vi "SeCrTs-Drive_Read_L.vi"(8 "error in":errorcluster, 9 "Message Queue":refnum<queue>, 11 "Data FIFO Ref":T1) -> (0 "error out":errorcluster)   [LabVIEW 2022 SP3]
uses:
  RT Controls/SeCrTs-Data FIFO.ctl
  RT Support/SeCrTs-RT_Global_R.vi
panel:
  in  "TCP_Port_Bottom":u16=3000
  in  "TCP_Port_Top":u16=2000
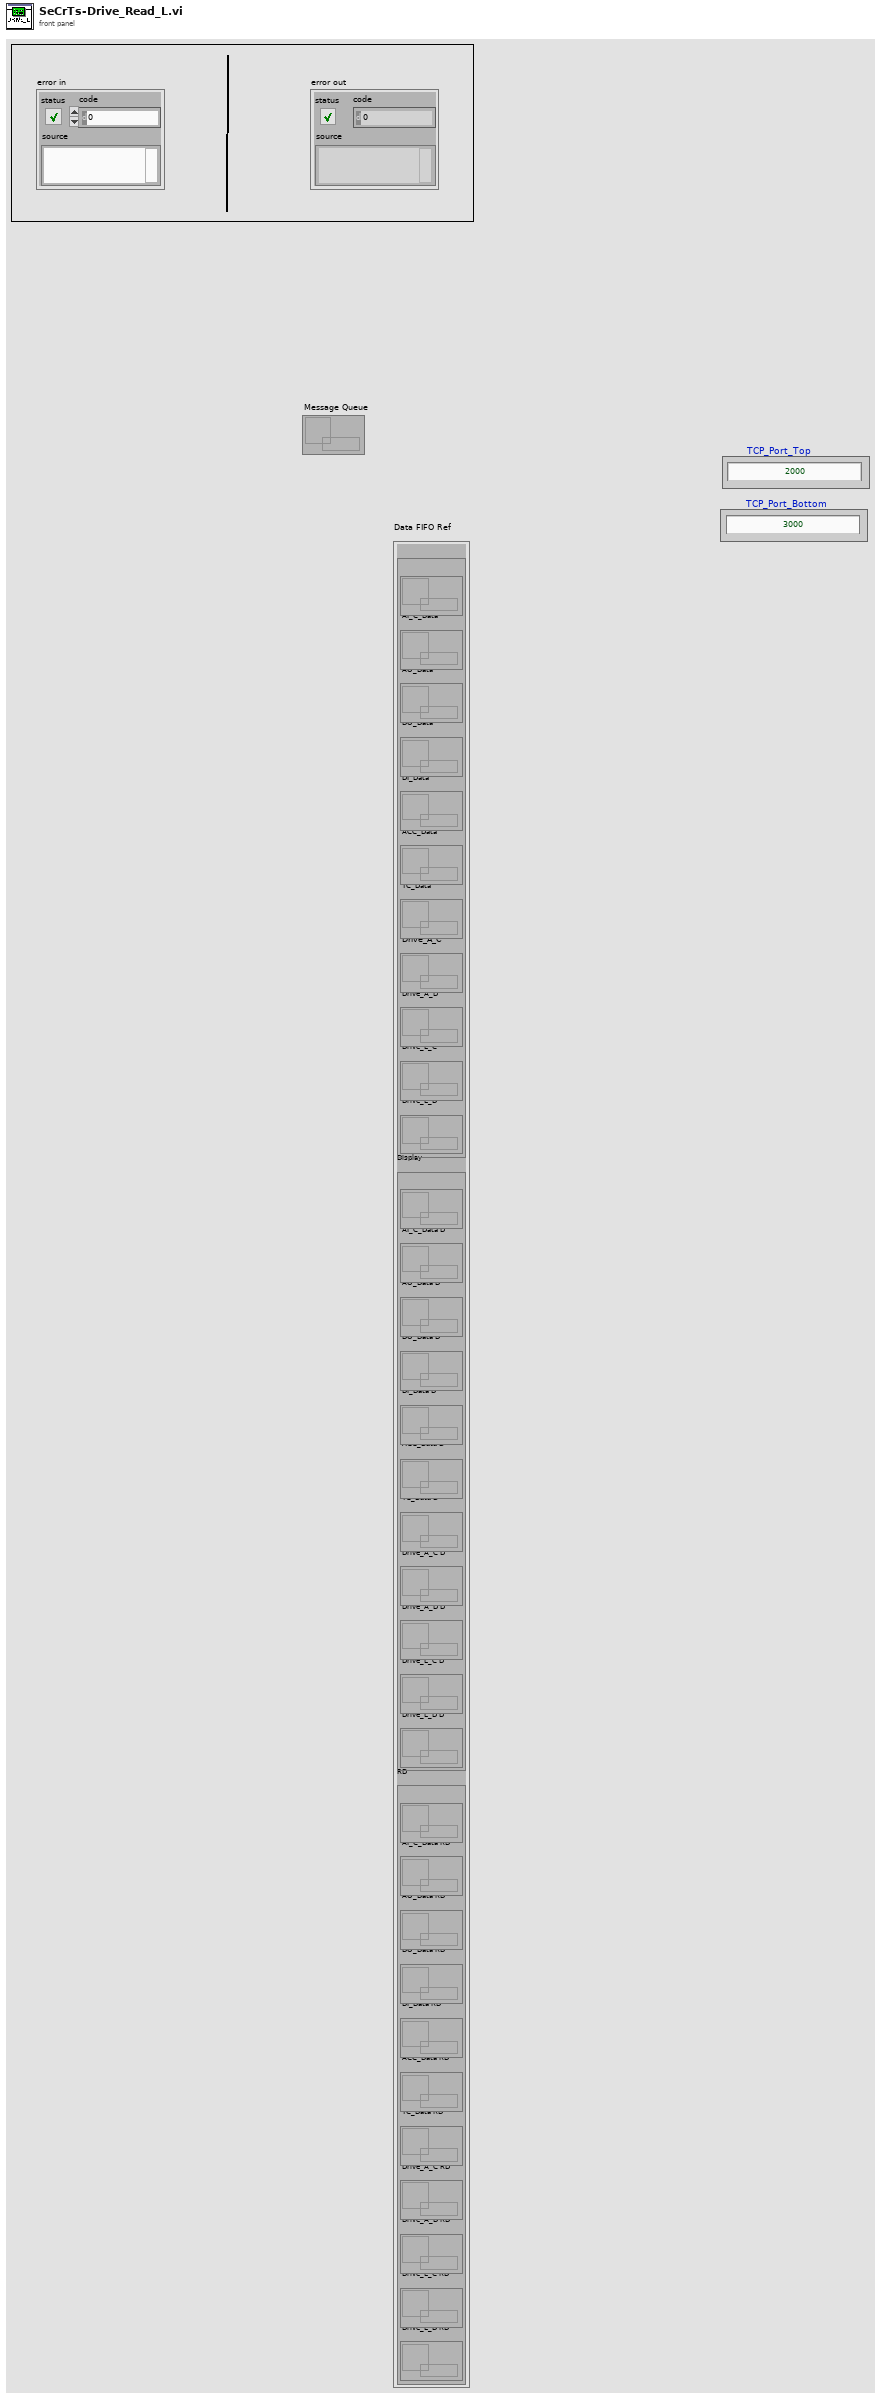
[diagram p1: front panel]
types:
  T1 = typedef "SeCrTs-Data FIFO.ctl" = cluster{"Control":cluster{"AI_V_Data":refnum<queue>, "AI_C_Data":refnum<queue>, "AO_Data":refnum<queue>, "DO_Data":refnum<queue>, "DI_Data":refnum<queue>, "ACC_Data":refnum<queue>, "TC_Data":refnum<queue>, "Drive_A_C":refnum<queue>, "Drive_A_D":refnum<queue>, "Drive_L_C":refnum<queue>, "Drive_L_D":refnum<queue>}, "Display":cluster{"AI_V_Data D":refnum<queue>, "AI_C_Data D":refnum<queue>, "AO_Data D":refnum<queue>, "DO_Data D":refnum<queue>, "DI_Data D":refnum<queue>, "ACC_Data D":refnum<queue>, "TC_Data D":refnum<queue>, "Drive_A_C D":refnum<queue>, "Drive_A_D D":refnum<queue>, "Drive_L_C D":refnum<queue>, "Drive_L_D D":refnum<queue>}, "RD":cluster{"AI_V_Data RD":refnum<queue>, "AI_C_Data RD":refnum<queue>, "AO_Data RD":refnum<queue>, "DO_Data RD":refnum<queue>, "DI_Data RD":refnum<queue>, "ACC_Data RD":refnum<queue>, "TC_Data RD":refnum<queue>, "Drive_A_C RD":refnum<queue>, "Drive_A_D RD":refnum<queue>, "Drive_L_C RD":refnum<queue>, "Drive_L_D RD":refnum<queue>}}
  T2 = enum16{"AI C", "AI V", "AO", "DI", "DO", "TC", "ACC", "DR L", "DR A"}
  T3 = enum16{"Init", "Read 'All'", "Read 'n'", "Read '1'", "Write '1'", "Write 'n'", "Write 'All'"}
  T4 = cluster{"Start DAQ":bool, "Stop DAQ":bool, "RT Stop":bool, "RT Exit":bool, "Start Seq":bool}
  T5 = cluster{"En_Drive_A":bool, "En_Drive_L":bool, "Exit_Drive_A":bool, "Exit_Drive_L":bool}
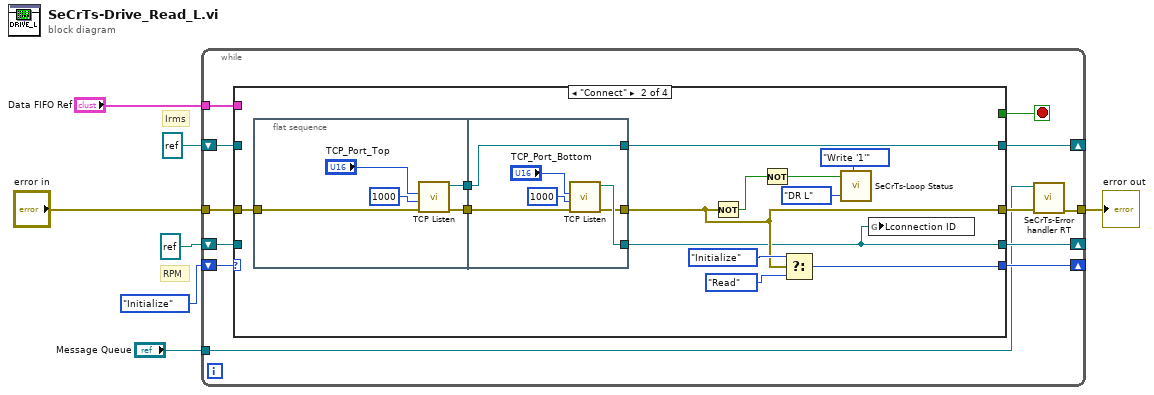
[diagram p0: block diagram]
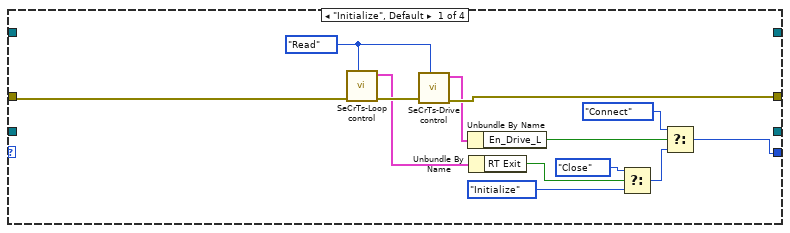
[diagram p2: hidden frame]
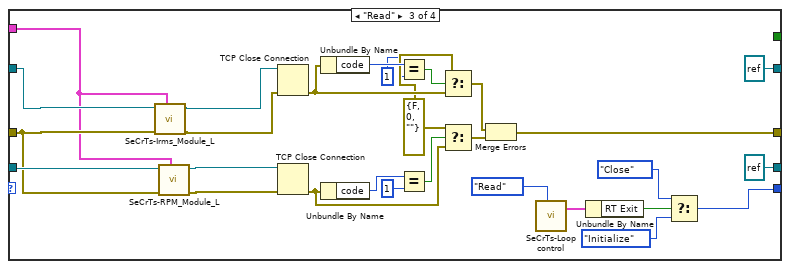
[diagram p3: hidden frame]
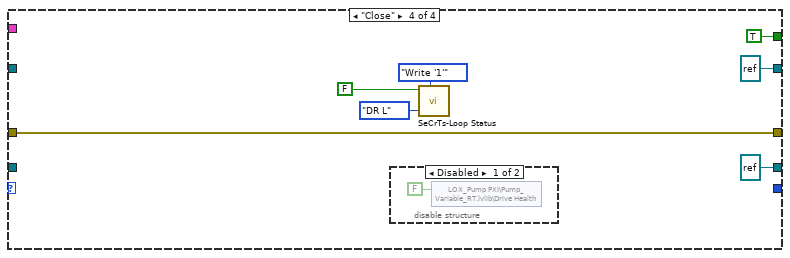
[diagram p4: hidden frame]
diagram:
  # "RPM"
  # "Irms"
  n1 = while {
    shift-right: [w18] -> _
    shift-left: enum16{"Initialize", "Connect", "Read", "Close"}."Initialize" -> [w19]
    tunnel: "error in" -> [w17]
    tunnel: [w9] -> w5
    shift-right: [w16] -> _
    shift-left: refnum<k5> refnum ("connection ID") -> [w14]
    shift-right: [w15] -> _
    shift-left: refnum<k5> refnum ("connection ID") -> [w13]
    tunnel: "Data FIFO Ref" -> [w11]
    tunnel: "Message Queue" -> [w8]
    stop <- w12 stop-if-true
    n2 = case shown="\"Connect\"" w19 {
      tunnel: [w32 w39 w82 _] -> w18
      tunnel: w17 -> [w27 w43 w59 w88]
      tunnel: [w25 w38 w70 w88] -> w10
      tunnel: [_ w42 refnum<k5> refnum ("TCP Network Connection out") refnum<k5> refnum ("TCP Network Connection out")] -> w16
      tunnel: [_ w37 refnum<k5> refnum ("TCP Network Connection out") refnum<k5> refnum ("TCP Network Connection out")] -> w15
      tunnel: w14 -> [_ _ w64 _]
      tunnel: w13 -> [_ _ w60 _]
      tunnel: [_ _ _ TRUE] -> w12
      tunnel: w11 -> [_ _ w57 _]
      frame "Initialize", Default {
        w24 = enum16{"Init", "Write", "Read"}."Read" ("Action")
        n3 = call "SeCrTs-Loop control.vi"("Action"=w24, "error in (no error)"=w27) -> ("error Out"=w26:errorcluster, "Loop Control out"=w23:T4)  [unwired: 8 in]
        n4 = call "SeCrTs-Drive control.vi"("Action"=w24, "error in"=w26) -> ("error Out"=w25:errorcluster, "Loop Control Out"=w21:T5)  [unwired: 8 in]
        n5 = Unbundle By Name(w21) -> ("En_Drive_L"=w20:bool)
        n6 = Unbundle By Name(w23) -> ("RT Exit"=w22:bool)
        n7 = Select(t=enum16{"Initialize", "Connect", "Read", "Close"}."Close", s=w22, f=enum16{"Initialize", "Connect", "Read", "Close"}."Initialize") -> (s? t:f=w28:enum16{"Initialize", "Connect", "Read", "Close"})
        n8 = Select(t=enum16{"Initialize", "Connect", "Read", "Close"}."Connect", s=w20, f=w28) -> (s? t:f=w32:enum16{"Initialize", "Connect", "Read", "Close"})
      }
      frame "Connect" {
        n9 = flat-sequence {
          tunnel: w43 -> [w48]
          tunnel: [w47] -> w45
          tunnel: [w46] -> w44
          tunnel: [w56] -> w37
          tunnel: w45 -> [w52]
          tunnel: w44 -> [w55]
          tunnel: [w55] -> w42
          tunnel: [w51] -> w38
          frame #0 {
            n10 = call <vilib>:"TCP Listen.vi"("error in (no error)"=w48, "timeout ms (wait forever: -1)"=1000, "port"="TCP_Port_Top") -> ("error out"=w47:errorcluster, "connection ID"=w46:refnum<k5>)  [unwired: 4 in, 3 out]
          }
          frame #1 {
            n11 = call <vilib>:"TCP Listen.vi"("error in (no error)"=w52, "timeout ms (wait forever: -1)"=1000, "port"="TCP_Port_Bottom") -> ("error out"=w51:errorcluster, "connection ID"=w56:refnum<k5>)  [unwired: 4 in, 3 out]
          }
        }
        n12 = Not(x=w38) -> (.not. x?=w33:bool)
        n13 = Not(x=w33) -> (.not. x?=w35:bool)
        n14 = Select(t=enum16{"Initialize", "Connect", "Read", "Close"}."Initialize", s=w38, f=enum16{"Initialize", "Connect", "Read", "Close"}."Read") -> (s? t:f=w39:enum16{"Initialize", "Connect", "Read", "Close"})
        n15 = call "SeCrTs-Loop Status.vi"("Option"=T3."Write '1'", "Status"=w35, "Loop"=T2."DR L") -> ()  [unwired: 6 in, 3 out]
        n16 = global write "SeCrTs-RT_Global_R.vi" "Lconnection ID"(w37) -> ()
      }
      frame "Read" {
        w73 = errorcluster {"status"=FALSE, "code"=0, "source"=""} ("error constant")
        n17 = call "SeCrTs-Irms_Module_L.vi"("Data FIFO Ref"=w57, "error in"=w59, "TCP Network Connection in"=w64) -> ("error out"=w63:errorcluster, "TCP Network Connection out"=w65:refnum<k5>)  [unwired: 7 in]
        n18 = call "SeCrTs-RPM_Module_L.vi"("Data FIFO Ref"=w57, "error in (no error)"=w59, "TCP Network Connection in"=w60) -> ("error out"=w62:errorcluster, "TCP Network Connection out"=w61:refnum<k5>)  [unwired: 7 in]
        n19 = TCP Close Connection(connection ID=w65, error in (no error)=w63) -> (error out=w77:errorcluster)  [unwired: 1 in, 1 out]
        n20 = TCP Close Connection(connection ID=w61, error in (no error)=w62) -> (error out=w76:errorcluster)  [unwired: 1 in, 1 out]
        n21 = Unbundle By Name(w77) -> ("code"=w81:i32)
        n22 = Unbundle By Name(w76) -> ("code"=w80:i32)
        n23 = Equal?(x=w81, y=1) -> (x = y?=w78:bool)
        n24 = Equal?(x=w80, y=1) -> (x = y?=w79:bool)
        n25 = Select(t=w73, s=w78, f=w77) -> (s? t:f=w75:errorcluster)
        n26 = Select(t=w73, s=w79, f=w76) -> (s? t:f=w74:errorcluster)
        n27 = Merge Errors(w75, w74) -> (w70:errorcluster)
        n28 = call "SeCrTs-Loop control.vi"("Action"=enum16{"Init", "Write", "Read"}."Read") -> ("Loop Control out"=w67:T4)  [unwired: 9 in, 1 out]
        n29 = Unbundle By Name(w67) -> ("RT Exit"=w66:bool)
        n30 = Select(t=enum16{"Initialize", "Connect", "Read", "Close"}."Close", s=w66, f=enum16{"Initialize", "Connect", "Read", "Close"}."Initialize") -> (s? t:f=w82:enum16{"Initialize", "Connect", "Read", "Close"})
      }
      frame "Close" {
        n31 = disable-structure shown="Disabled" {
          frame Disabled {
            n32 = shared-variable "LOX_Pump PXI\\Pump_Variable_RT.lvlib\\Drive Health"(FALSE ("Drive Health")) -> ()  [unwired: 1 in, 1 out]
          }
          frame Enabled {
          }
        }
        n33 = call "SeCrTs-Loop Status.vi"("Option"=T3."Write '1'", "Status"=FALSE, "Loop"=T2."DR L") -> ()  [unwired: 6 in, 3 out]
      }
    }
    n34 = call "SeCrTs-Error handler RT.vi"("error in"=w10, "Message Queue"=w8) -> ("error out"=w9:errorcluster)  [unwired: 8 in, 1 out]
  }
  "error out" <- w5
